vi "Agilent DMM Trigger and Fetch.vi"(8 "error in (no error)":errorcluster, 10 "Timeout (10000ms)":u32=10000, 11 "VISA Resource Name":refnum<visa-resource-name>) -> (0 "error out":errorcluster, 2 "Data Reading":T1 caption="This reading is allways in the base units\ni.e. V, A, Ohms, Hz, Sec, etc." format="%#_10f", 3 "dup VISA Resource Name":refnum<visa-resource-name>)   [LabVIEW 2011]
doc: "This VI for the HP 8753 is used to read the sweep type.\n\n0 LINEAR FREQ\n1 LOG FREQ\n2 LIST FREQ\n3 CW TIME\n4 POWER SWEEP"
uses:
  DMM Measurement.ctl
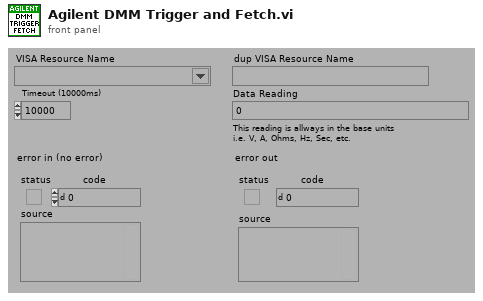
[diagram p1: front panel]
types:
  T1 = typedef "DMM Measurement.ctl" = dbl
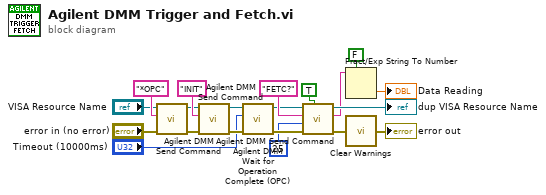
[diagram p0: block diagram]
diagram:
  n1 = call "Agilent DMM Send Command.vi"("error in (no error)"="error in (no error)", "Command"="*OPC" ("write buffer"), "VISA Resource Name"="VISA Resource Name") -> ("error out"=w7:errorcluster, "dup VISA Resource Name"=w8:refnum<visa-resource-name>)  [unwired: 2 in, 5 out]
  n2 = call "Agilent DMM Send Command.vi"("error in (no error)"=w7, "Command"="INIT" ("write buffer"), "VISA Resource Name"=w8) -> ("error out"=w16:errorcluster, "dup VISA Resource Name"=w13:refnum<visa-resource-name>)  [unwired: 2 in, 5 out]
  n3 = call "Agilent DMM Wait for Operation Complete (OPC).vi"("error in (no error)"=w16, "Timeout, ms (10000)"="Timeout (10000ms)", "VISA Resource Name"=w13) -> ("error out"=w15:errorcluster, "dup VISA Resource Name"=w14:refnum<visa-resource-name>)  [unwired: 7 out]
  n4 = call "Agilent DMM Send Command.vi"("Read? (F)"=TRUE, "error in (no error)"=w15, "Byte Count"=u32 25 ("byte count"), "Command"="FETC?" ("write buffer"), "VISA Resource Name"=w14) -> ("error out"=w4:errorcluster, "Data Read"=w3:string, "dup VISA Resource Name"=→"dup VISA Resource Name":refnum<visa-resource-name>)  [unwired: 4 out]
  n5 = Fract/Exp String To Number(use system decimal point (T)=FALSE, string=w3) -> (number=→"Data Reading":dbl)  [unwired: 3 out]
  n6 = call "Clear Warnings.vi"("error in (no error)"=w4) -> ("error out"=→"error out":errorcluster)
